vi "SECADO_enterEnsayo.vi"(8 "error in (no error)":errorcluster) -> (0 "error out":errorcluster, 1 "Datos.Lecho":T1={"Clasificacion"="Grueso (2,5<Dp<4", "Masa, g"=500.0, "Altura, cm"=45.0, "Diam_part, mm"=5.0, "Dens_part, g/cm3"=1.0, "Hum_ini, f1"=60.0, "Temp_ini, C"=25.0} {"Hum_ini, f1" format="%.2f"; "Temp_ini, C" format="%.2f"; "Masa, g" format="%.2f"; "Altura, cm" format="%.2f"; "Diam_part, mm" format="%.2f"; "Dens_part, g/cm3" format="%.2f"}, 2 "Constantes.Ensayo":T2={"Num.Ensayo"=0, "Diam_reactor, cm"=0.0, "Resistencia, ohm"=50.0, "Voltaje_resist, vac"=0.0, "Hum_ext, f1"=0.0, "Vel.min_fluido, m/s"=0.0, "Vel_arrastre, m/s"=10.0, "SET Caudal_vent, g/s"=0.0} {"Vel_arrastre, m/s" format="%.2f"; "SET Caudal_vent, g/s" format="%.2f"; "Diam_reactor, cm" format="%.2f"; "Resistencia, ohm" format="%.2f"; "Voltaje_resist, vac" format="%.2f"; "Hum_ext, f1" format="%.2f"; "Vel.min_fluido, m/s" format="%.2f"}, 5 "Cancelled?":bool)   [LabVIEW 2017]
doc: "Use this template to create a dialog box with event handling."
uses:
  Typedefs/SECADO_constantes.Ensayo--Cluster.ctl
  Typedefs/SECADO_datos.Lecho--Cluster.ctl
panel:
  in  "SET Caudal_vent, g/s":dbl format="%.2f"
  in  "Hum_ini, f1":dbl=0.6 format="%.2f"
  in  "Temp_ini, C":dbl=25.0 format="%.2f"
  in  "Masa, g":dbl=500.0 format="%.2f"
  in  "Altura, cm":dbl=45.0 format="%.2f"
  in  "Diam_part, mm":dbl=5.0 format="%.2f"
  in  "Dens_part, g/cm3":dbl=1.0 format="%.2f"
  in  "Clasificacion":string="Grueso (2,5<Dp<4"
  in  "Vel_arrastre, m/s":dbl=10.0 format="%.2f"
  in  "Num.Ensayo":i32=1
  in  "Diam_reactor, cm":dbl=20.0 format="%.2f"
  in  "Resistencia, ohm":dbl=50.0 format="%.2f"
  in  "Voltaje_resist, vac":dbl=230.0 format="%.2f"
  in  "Hum_ext, f1":dbl=0.6 format="%.2f"
  in  "Vel.min_fluido, m/s":dbl=1.0 format="%.2f"
  out "Hora":string
  out "Fecha":string
  in  "Cancel":bool
  in  "OK":bool
  # "Datos del ensayo"
  # "( Introduce los datos que aparecen en color azul )"
  # "Constantes.Ensayo"
  # "Datos.Lecho"
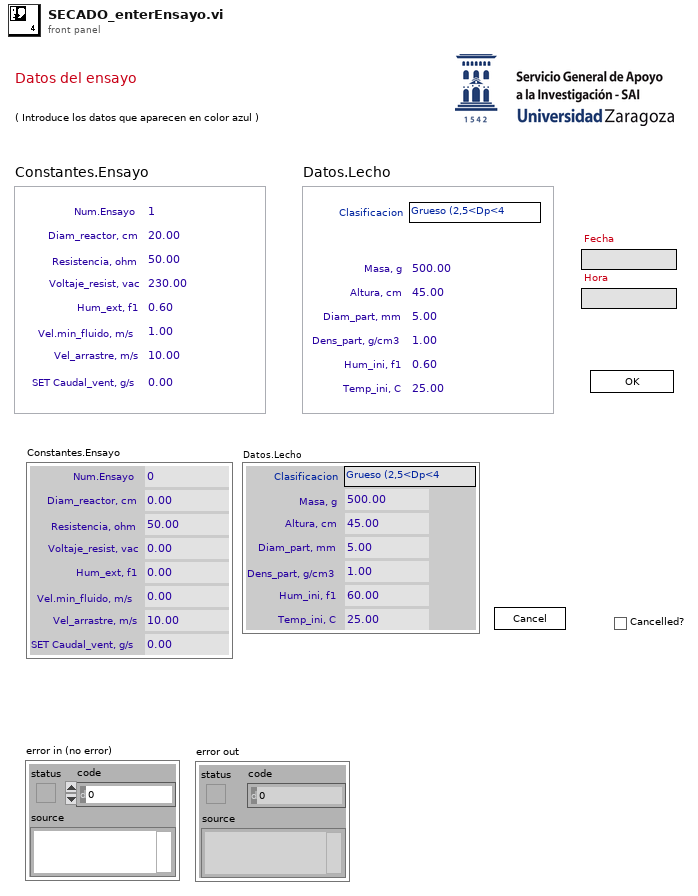
[diagram p1: front panel]
types:
  T1 = typedef "SECADO_datos.Lecho--Cluster.ctl" = cluster{"Clasificacion":string, "Masa, g":dbl, "Altura, cm":dbl, "Diam_part, mm":dbl, "Dens_part, g/cm3":dbl, "Hum_ini, f1":dbl, "Temp_ini, C":dbl}
  T2 = typedef "SECADO_constantes.Ensayo--Cluster.ctl" = cluster{"Num.Ensayo":i32, "Diam_reactor, cm":dbl, "Resistencia, ohm":dbl, "Voltaje_resist, vac":dbl, "Hum_ext, f1":dbl, "Vel.min_fluido, m/s":dbl, "Vel_arrastre, m/s":dbl, "SET Caudal_vent, g/s":dbl}
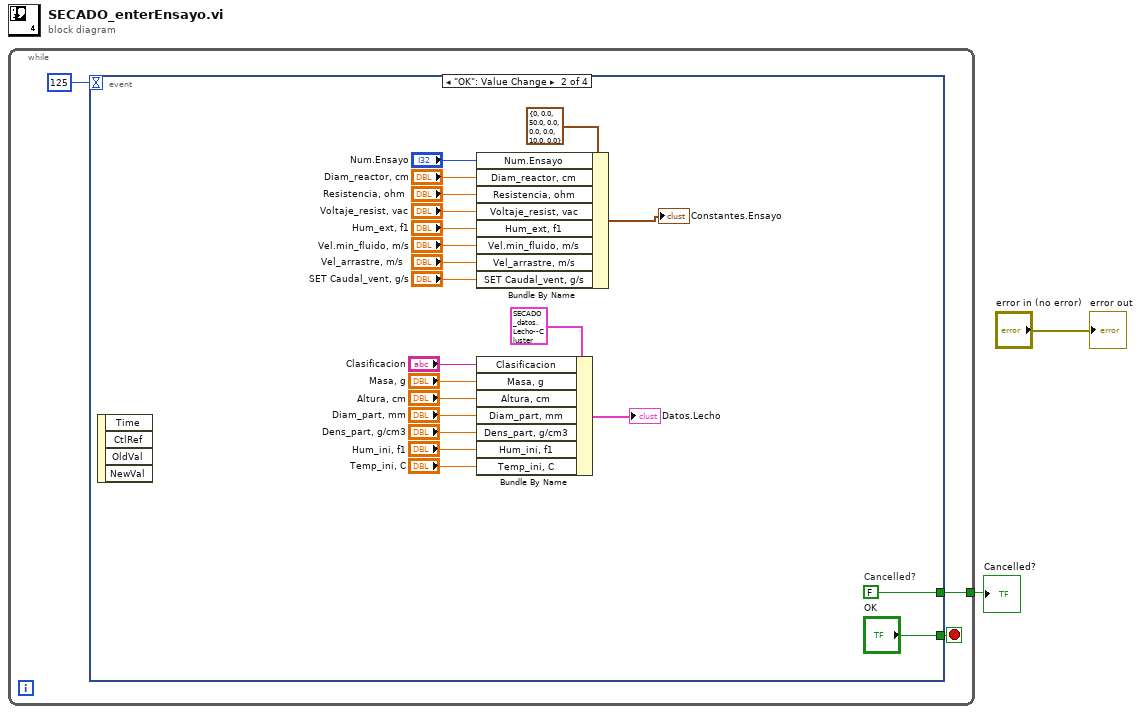
[diagram p0: block diagram]
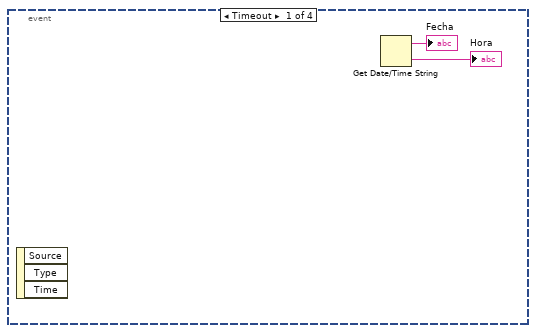
[diagram p2: hidden frame]
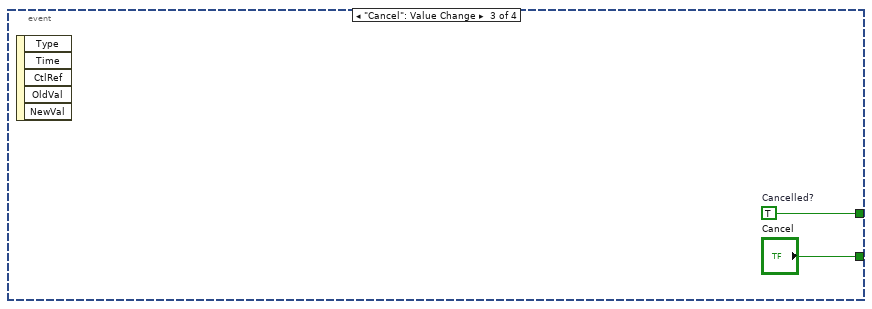
[diagram p3: hidden frame]
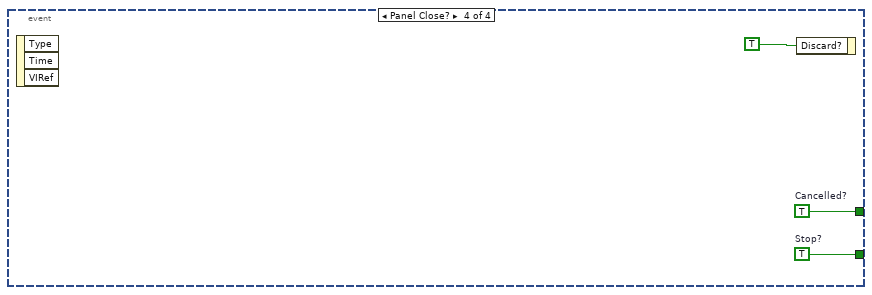
[diagram p4: hidden frame]
diagram:
  n1 = while {
    tunnel: [w4] -> w2
    stop <- w5 stop-if-true
    n2 = event shown="[1] \"OK\": Value Change" {
      selector: _ -> [_ _ _ _]
      dyn-events: _ -> [_ _ _ _]
      timeout: 125 -> [_ _ _ _]
      tunnel: [_ "OK" "Cancel" w32] -> w5
      tunnel: [_ w28 w30 w31] -> w4
      event Timeout {
        n3 = event-data() -> ()  [unwired: 1 in, 3 out]
        n4 = Get Date/Time String() -> (date string=→"Fecha":string, time string=→"Hora":string)  [unwired: 3 in]
      }
      event "OK": Value Change {
        w28 = FALSE  # Cancelled?
        n5 = event-data() -> ()  [unwired: 1 in, 4 out]
        n6 = Bundle By Name(cluster=T2 {"Num.Ensayo"=0, "Diam_reactor, cm"=0.0, "Resistencia, ohm"=50.0, "Voltaje_resist, vac"=0.0, "Hum_ext, f1"=0.0, "Vel.min_fluido, m/s"=0.0, "Vel_arrastre, m/s"=10.0, "SET Caudal_vent, g/s"=0.0} ("Window"), "Num.Ensayo"="Num.Ensayo", "Diam_reactor, cm"="Diam_reactor, cm", "Resistencia, ohm"="Resistencia, ohm", "Voltaje_resist, vac"="Voltaje_resist, vac", "Hum_ext, f1"="Hum_ext, f1", "Vel.min_fluido, m/s"="Vel.min_fluido, m/s", "Vel_arrastre, m/s"="Vel_arrastre, m/s", "SET Caudal_vent, g/s"="SET Caudal_vent, g/s") -> (→"Constantes.Ensayo":T2)
        n7 = Bundle By Name(cluster=T1 {"Clasificacion"="Grueso (2,5<Dp<4", "Masa, g"=500.0, "Altura, cm"=45.0, "Diam_part, mm"=5.0, "Dens_part, g/cm3"=1.0, "Hum_ini, f1"=60.0, "Temp_ini, C"=25.0} ("Datos.Lecho"), "Clasificacion"="Clasificacion", "Masa, g"="Masa, g", "Altura, cm"="Altura, cm", "Diam_part, mm"="Diam_part, mm", "Dens_part, g/cm3"="Dens_part, g/cm3", "Hum_ini, f1"="Hum_ini, f1", "Temp_ini, C"="Temp_ini, C") -> (→"Datos.Lecho":T1)
      }
      event "Cancel": Value Change {
        w30 = TRUE  # Cancelled?
        n8 = event-data() -> ()  [unwired: 1 in, 5 out]
      }
      event Panel Close? {
        w31 = TRUE  # Cancelled?
        w32 = TRUE  # Stop?
        n9 = event-data() -> ()  [unwired: 1 in, 3 out]
        n10 = event-data("Discard?"=TRUE) -> ()  [unwired: 1 in, 1 out]
      }
    }
  }
  "Cancelled?" <- w2
  "error out" <- "error in (no error)"
